vi "Read A.vi"(8 "error in (no error)":errorcluster, 11 "Linear in":refnum<class "Linear.lvclass">) -> (0 "error out":errorcluster, 2 "A":dbl, 3 "Linear out":refnum<class "Linear.lvclass">)   [LabVIEW 2020, in "Data Generators.lvlib" / "Linear.lvclass"]
uses:
  Linear.lvclass
  Linear.lvclass/Linear.ctl
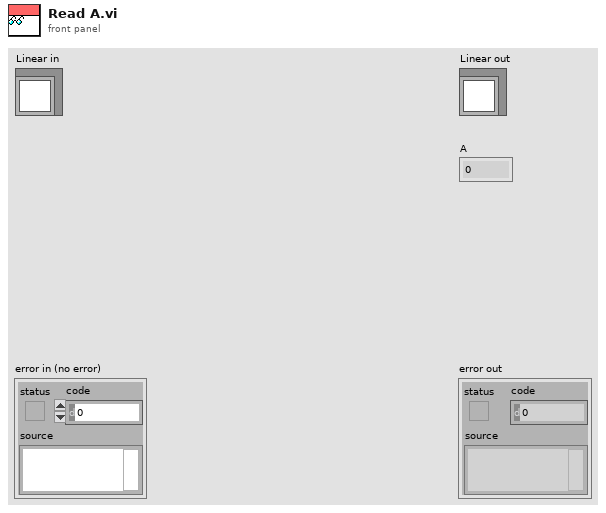
[diagram p1: front panel]
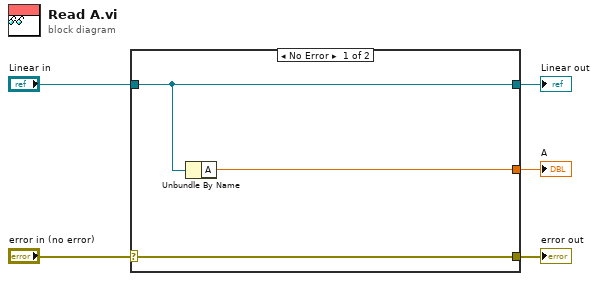
[diagram p0: block diagram]
diagram:
  n1 = case shown="No Error" "error in (no error)" {
    selector: "error in (no error)" -> [w8 w9]
    tunnel: [w8 w9] -> w4
    tunnel: [w7 w10] -> w2
    tunnel: "Linear in" -> [w7 w10]
    tunnel: [w6 _] -> w1
    frame No Error {
      n2 = Unbundle By Name(w7) -> ("A"=w6:dbl)
    }
    frame Error {
    }
  }
  "error out" <- w4
  "Linear out" <- w2
  "A" <- w1
